vi "Heater Status.vi"(8 "error in (no error)":errorcluster, 10 "Heater Output (1:1)":u16(ring)=1 items=["1"=1, "2"=2], 11 "VISA resource name":refnum<visa-resource-name>) -> (0 "error out":errorcluster, 2 "Heater Status":u16(ring) items=["No Error", "Heater Open Load", "Heater Short"], 3 "VISA resource name out":refnum<visa-resource-name>)   [LabVIEW 2012, in "Lake Shore 336.lvlib"]
doc: "This VI returns the Heater Output status. The output will be turned off in the event of an open or short circuit error condition. An error condition is cleared upon querying the heater status, which will also clear the front panel error message."
uses:
  Lake Shore 336.lvlib
  Instance           1 21Saved   Heater Status .vi
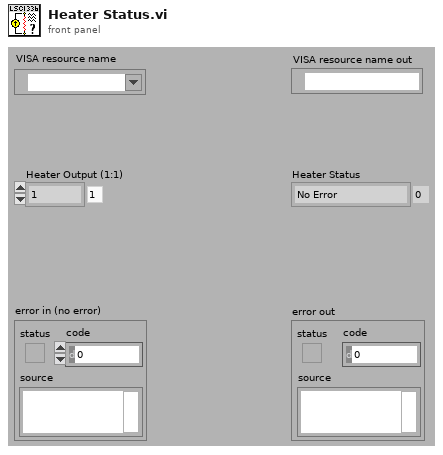
[diagram p1: front panel]
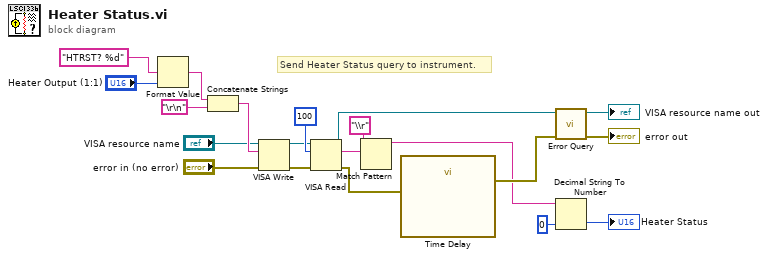
[diagram p0: block diagram]
diagram:
  # "Send Heater Status query to instrument."
  n1 = Format Value(format string="HTRST? %d", value (0)="Heater Output (1:1)") -> (output string=w1:string)  [unwired: 1 in]
  n2 = Concatenate Strings(w1, "\r\n") -> (w9:string)
  n3 = VISA Write(VISA resource name="VISA resource name", write buffer=w9, error in (no error)="error in (no error)") -> (VISA resource name out=w13:refnum<visa-resource-name>, error out=w12:errorcluster)  [unwired: 1 out]
  n4 = VISA Read(VISA resource name=w13, byte count=100, error in (no error)=w12) -> (VISA resource name out=w7:refnum<visa-resource-name>, read buffer=w15:string, error out=w11:errorcluster)  [unwired: 1 out]
  n5 = Match Pattern(string=w15, regular expression="\\r") -> (before substring=w6:string)  [unwired: 1 in, 3 out]
  n6 = call "Time Delay"("error in (no error)"=w11) -> ("error out"=w8:errorcluster)  [unwired: 10 in]
  n7 = call "Error Query.vi"("error in (no error)"=w8, "VISA resource name"=w7) -> ("error out"=→"error out":errorcluster, "VISA resource name out"=→"VISA resource name out":refnum<visa-resource-name>)  [unwired: 7 in, 1 out]
  n8 = Decimal String To Number(string=w6, default (0L)=u16 0) -> (number=→"Heater Status":u16)  [unwired: 1 in, 1 out]
